vi "2D scan tiled.vi"(6 "WatchDog Mode":u16(ring)=2 items=["Do Nothing", "Send Idle Only", "Watch FIB & SEM", "Watch FIB Only", "Watch SEM Only"], 10 "Tiled scan inputs":T6={"HW Config"={"SEM X coil"="SEM-X", "SEM Y coil"="SEM-Y", "Detectors"="Detectors", "Det min (V)"=-10.0, "Det max (V)"=10.0, "Eanable COM"=TRUE, "COM port"="COM1", "Detector FIB-NI auto switch"="FIB/port0/line0", "Machine Type"=0, "Machine ID"="Feiss/Sigma-01-42", "SEM Max FOV (um)"=350.0}, "Det Info"={"Brightness A"=40.0, "Contrast A"=26.0, "Detector B name"="ESB @ 1.0 kV", "Brightness B"=40.0, "Contrast B"=40.0, "Detector C name"="PMT @ 6.0", "Detector D name"="Detector D"}, "SEM Scan Parameters"={"X size (um)"=20.0, "Y size (um)"=20.0, "X center (um)"=0.0, "Y center (um)"=0.0, "X size (V)"=6.190428211586902, "X size auto"=TRUE, "X stig"=[[0.0]], "Y stig"=[[0.0]], "X aln"=[[0.0]], "Y aln"=[[0.0]], "Scan rate (Hz)"=10000000, "Oversampling"=5, "Oversampling auto"=TRUE, "Frame line rampdown ratio"=0.1, "Pixel size (nm)"=10.0, "WD (mm)"=[[3.0]], "X tiles"=1, "Y tiles"=1, "Overlap (um)"=1.0, "Interlaced"=TRUE, "dX (um)"=[0.0], "dY (um)"=[0.0], "Frames"=1}, "SEM Options"={"GetInfo"=TRUE, "Set Det A para"=TRUE, "Set WD"=FALSE, "Set Mag"=TRUE, "Set stig"=FALSE, "Set aln"=FALSE, "Display"=TRUE, "Save"=TRUE, "8-bit"=TRUE, "Detector A"=TRUE, "Detector B"=FALSE, "Detector C"=FALSE, "Detector D"=FALSE, "Inverse A"=FALSE, "Inverse B"=FALSE, "Inverse C"=FALSE, "Inverse D"=FALSE, "Inverse PNG"=TRUE, "Freeze"=TRUE, "PNG only"=FALSE, "Upload"=FALSE, "Delete after upload"=FALSE}, "Focus Index Options"={"Keep aspect ratio"=FALSE, "Show Focus Index"=TRUE, "Focus Index primary grid center"=TRUE, "X Grids"=[[0]], "Y Grids"=[[0]], "Primary X index"=[[0]], "Primary Y index"=[[0]]}, "File Information"={"File path"=path "E:/Images", "Notes"="", "Save recipe"=FALSE, "Load recipe"=FALSE, "Sample ID"=""}, "Milling para"={"X resolution"=4096, "Y resolution"=125001, "X offset (um)"=0.0, "Y offset (um)"=0.0, "X center (um)"=0.0, "Y center (um)"=0.0, "X size (um)"=250.0, "Y size (um)"=250.0, "UL-Ang"=90.0, "UR-Ang"=90.0, "Line milling time (s)"=5.0, "Z-step (nm)"=2.0, "Lines auto pause"=1, "Auto pause"=FALSE, "Mill from Bottom"=FALSE, "FIB FOV (um)"=500.0, "Auto Profile"=FALSE, "Mill start from Last"=FALSE, "FIB PID on"=FALSE, "FIB PID reset"=TRUE, "FIB PID measured"=0, "FIB PID target"=0.0, "FIB PID target slope"=0.0, "FIB PID P"=0.001, "FIB PID I"=0.01, "FIB PID D"=0.0, "Emission (uA)"=1.36, "Suppressor (V)"=50.0, "Auto reheat"=FALSE}, "Additional Info"={"Restart flag"=0, "Stage move flag"=0}} {"Milling para"."Suppressor (V)" step=0.1 format="%.1g"; "Milling para"."Emission (uA)" step=0.1 format="%.2g"; "Milling para"."FIB PID measured" items=["Spec.", "B.D. 1", "B.D. 2", "Mill", "Spec. +"]; "Milling para"."FIB PID target slope" min=-1 max=1 step=0.1; "Milling para"."UR-Ang" format="%.2f"; "Milling para"."UL-Ang" format="%.2f"; "Milling para"."Y offset (um)" step=0.02 format="%.3g"; "Milling para"."X offset (um)" step=1 format="%.3g"; "Milling para"."FIB FOV (um)" format="%.3g"; "Milling para"."Line milling time (s)" format="%.1f"; "Milling para"."Y center (um)" format="%#.3g"; "Milling para"."X center (um)" format="%#.3g"; "SEM Scan Parameters"."dY (um)" format="%.1f"; "SEM Scan Parameters"."dX (um)" format="%.1f"; "SEM Scan Parameters"."Frames" min=1 step=1; "SEM Scan Parameters"."WD (mm)" format="%.1f"; "SEM Scan Parameters"."Y aln" format="%.1f"; "SEM Scan Parameters"."X aln" format="%.1f"; "SEM Scan Parameters"."Y stig" format="%.1f"; "SEM Scan Parameters"."X stig" format="%.1f"; "SEM Scan Parameters"."Overlap (um)" min=0; "SEM Scan Parameters"."Y tiles" min=1; "SEM Scan Parameters"."X tiles" min=1; "SEM Scan Parameters"."X size (um)" format="%.2f"; "SEM Scan Parameters"."Y size (um)" format="%.2f"; "SEM Scan Parameters"."Frame line rampdown ratio" min=0 max=1 step=0.05 format="%.2g"; "SEM Scan Parameters"."X center (um)" step=1 format="%.2f"; "SEM Scan Parameters"."Y center (um)" step=1 format="%.2f"; "SEM Scan Parameters"."X size (V)" format="%_4g"; "SEM Scan Parameters"."Scan rate (Hz)" max=4000000 step=100000 format="%.2e"; "HW Config"."Machine Type" items=["Feiss", "NVision"]}, 11 "ActiveX Container":refnum<k7>(container)) -> (0 "Image Focus Index Tiled":T3, 1 "Image Focus Index Array Tiled":T2, 2 "Low res scale Tiled (um/pix)":dbl[][](array[numeric]), 3 "Single scan outputs":T4={"SEM Status"={"AO SampClk.MaxRate"=100000000.0, "AI SampClk.MaxRate"=100000000.0, "AO rate"=10000000.0, "Scan speed"=1, "Detector #"=1, "X min (V)"=-3.095214105793451, "X max (V)"=3.095214105793451, "X min index"=0, "X max index"=1999, "AO multiline"=64, "Decimating factor"=3, "AvailSampPerChan"=832704, "AO scan line"=2000, "Total pixels recorded"=4096000, "Lines scanned"=2000, "Scan time (m)"=0.0, "Scan time (s)"=0.4416, "Remaining time (m)"=0, "Remaining time (s)"=0, "SEM Spec. I (nA)"=0.0, "Frame"=1, "X tile"=1, "Y tile"=1}, "SEM Parameters"={"Detector A"="InLens", "Detector B"="ESB @ 1.0 kV", "Brightness A"=40.0, "Contrast A"=26.0, "Brightness B"=40.0, "Contrast B"=40.0, "Magnification"=1769.4047, "Pixel size"=3.9210947, "Working distance"=2.91745, "EHT"=0.6, "Aperture"=1, "High current mode"=1, "Probe current"=613.0, "Scan rotation"=260.0, "Chamber vac"=1.43287e-06, "Gun vac"=3.9272e-10, "Beam shift X"=0.0, "Beam shift Y"=0.0, "Stig X"=-4.213583, "Stig Y"=-1.875912, "Alignment X"=1.861752, "Alignment Y"=-2.407838, "Stage X"=68.4182, "Stage Y"=64.91782, "Stage Z"=32.8349, "Stage T"=0.0, "Stage R"=153.14406, "Stage M"=0.0}, "Image Focus Index"={"A Img Focus Index"=0.014358657, "B Img Focus Index"=0.0, "C Img Focus Index"=0.0, "D Img Focus Index"=0.0}, "FIB parameters"={"FIB mode"=0, "FIB focus"=0.0, "FIB probe current"=0.0, "FIB emission current"=0.0, "FIB rotation"=0.0, "FIB aperture X"=0.0, "FIB aperture Y"=0.0, "FIB stig X"=0.0, "FIB stig Y"=0.0, "FIB beam shift X"=0.0, "FIB beam shift Y"=0.0}, "Image Focus Index Array"={"A Img Focus Index array"=[[0.014358657]], "B Img Focus Index array"=[], "C Img Focus Index array"=[], "D Img Focus Index array"=[]}} {"SEM Status"."Frame" min=1 step=1; "SEM Status"."Y tile" min=1; "SEM Status"."X tile" min=1; "SEM Status"."SEM Spec. I (nA)" format="%.2g"; "SEM Status"."AvailSampPerChan" scale=0.0..32000000.0; "SEM Status"."Scan time (s)" format="%.3f"; "SEM Status"."Total pixels recorded" scale=-1.0..37748736.0; "SEM Status"."Scan speed" scale=1.0..15.0; "SEM Status"."AO rate" format="%#_3e"}, 4 "SEM Spec. I Tiled (nA)":sgl[][](array[numeric]), 5 "8-bit over scale":bool[](array[boolean]))   [LabVIEW 2018]
uses:
  <vilib>/Analysis/baseanly.llb/Mean (DBL).vi
  <vilib>/Analysis/NI_AALBase.lvlib
panel:
  in  "Focus Index Options":T1={"Keep aspect ratio"=FALSE, "X Grids"=1, "Y Grids"=1, "Primary X index"=0, "Primary Y index"=0}
  out "Aln X Tiled":sgl[][](array[numeric])
  out "Aln Y Tiled":sgl[][](array[numeric])
  out "Stig Y Tiled":sgl[][](array[numeric])
  out "Stig X Tiled":sgl[][](array[numeric])
  out "WD Tiled":sgl[][](array[numeric])
  out "Det B Img Tiled":i16[][](graph)
  out "Det A Img Tiled":i16[][](graph)
  out "Tiled image Y index":u16[][](array[numeric])
  out "Tiled image X index":u16[][](array[numeric])
  out "Tiled image scale (um/pix)":sgl
  out "X size (V)":dbl[][](array[numeric])=[[2000.0]]
  out "Y center (um)":sgl[][](array[numeric])
  out "X center (um)":sgl[][](array[numeric])
  out "Y resolution":u32[][](array[numeric])=[[2000]]
  out "X resolution":u32[][](array[numeric])=[[2000]]
  in  "SEM Scan Parameters":T5={"X resolution"=6144, "Y resolution"=6144, "X center (um)"=0.0, "Y center (um)"=0.0, "X size (V)"=6.190428211586902, "X size auto"=TRUE, "X stig"=0.0, "Y stig"=0.0, "X aln"=0.0, "Y aln"=0.0, "Scan rate (Hz)"=10000000, "Oversampling"=5, "Oversampling auto"=TRUE, "Frame line rampdown ratio"=0.1, "Pixel size (nm)"=10.0, "WD (mm)"=0.0} {"Y aln" step=0.2 format="%.1g"; "X aln" step=0.2 format="%.1g"; "Y stig" step=0.2 format="%.1g"; "X stig" step=0.2 format="%.1g"; "WD (mm)" step=0.001 format="%.6g"; "Frame line rampdown ratio" min=0 max=1 step=0.05 format="%.2g"; "X center (um)" step=1.0 format="%.2f"; "Y center (um)" step=1.0 format="%.2f"; "X size (V)" format="%_4g"; "Scan rate (Hz)" max=4000000 step=100000 format="%.2e"}
  # "Hz"
  # "Scanning time"
  # "m"
  # "s"
  # "Remaining time"
  # "m"
  # "s"
  # "Direction"
  # "Start\nfrom"
  # "<"
  # "Grids"
  # "Primary"
  # "Recipe"
  # "Det"
  # "after"
  # "Detector A"
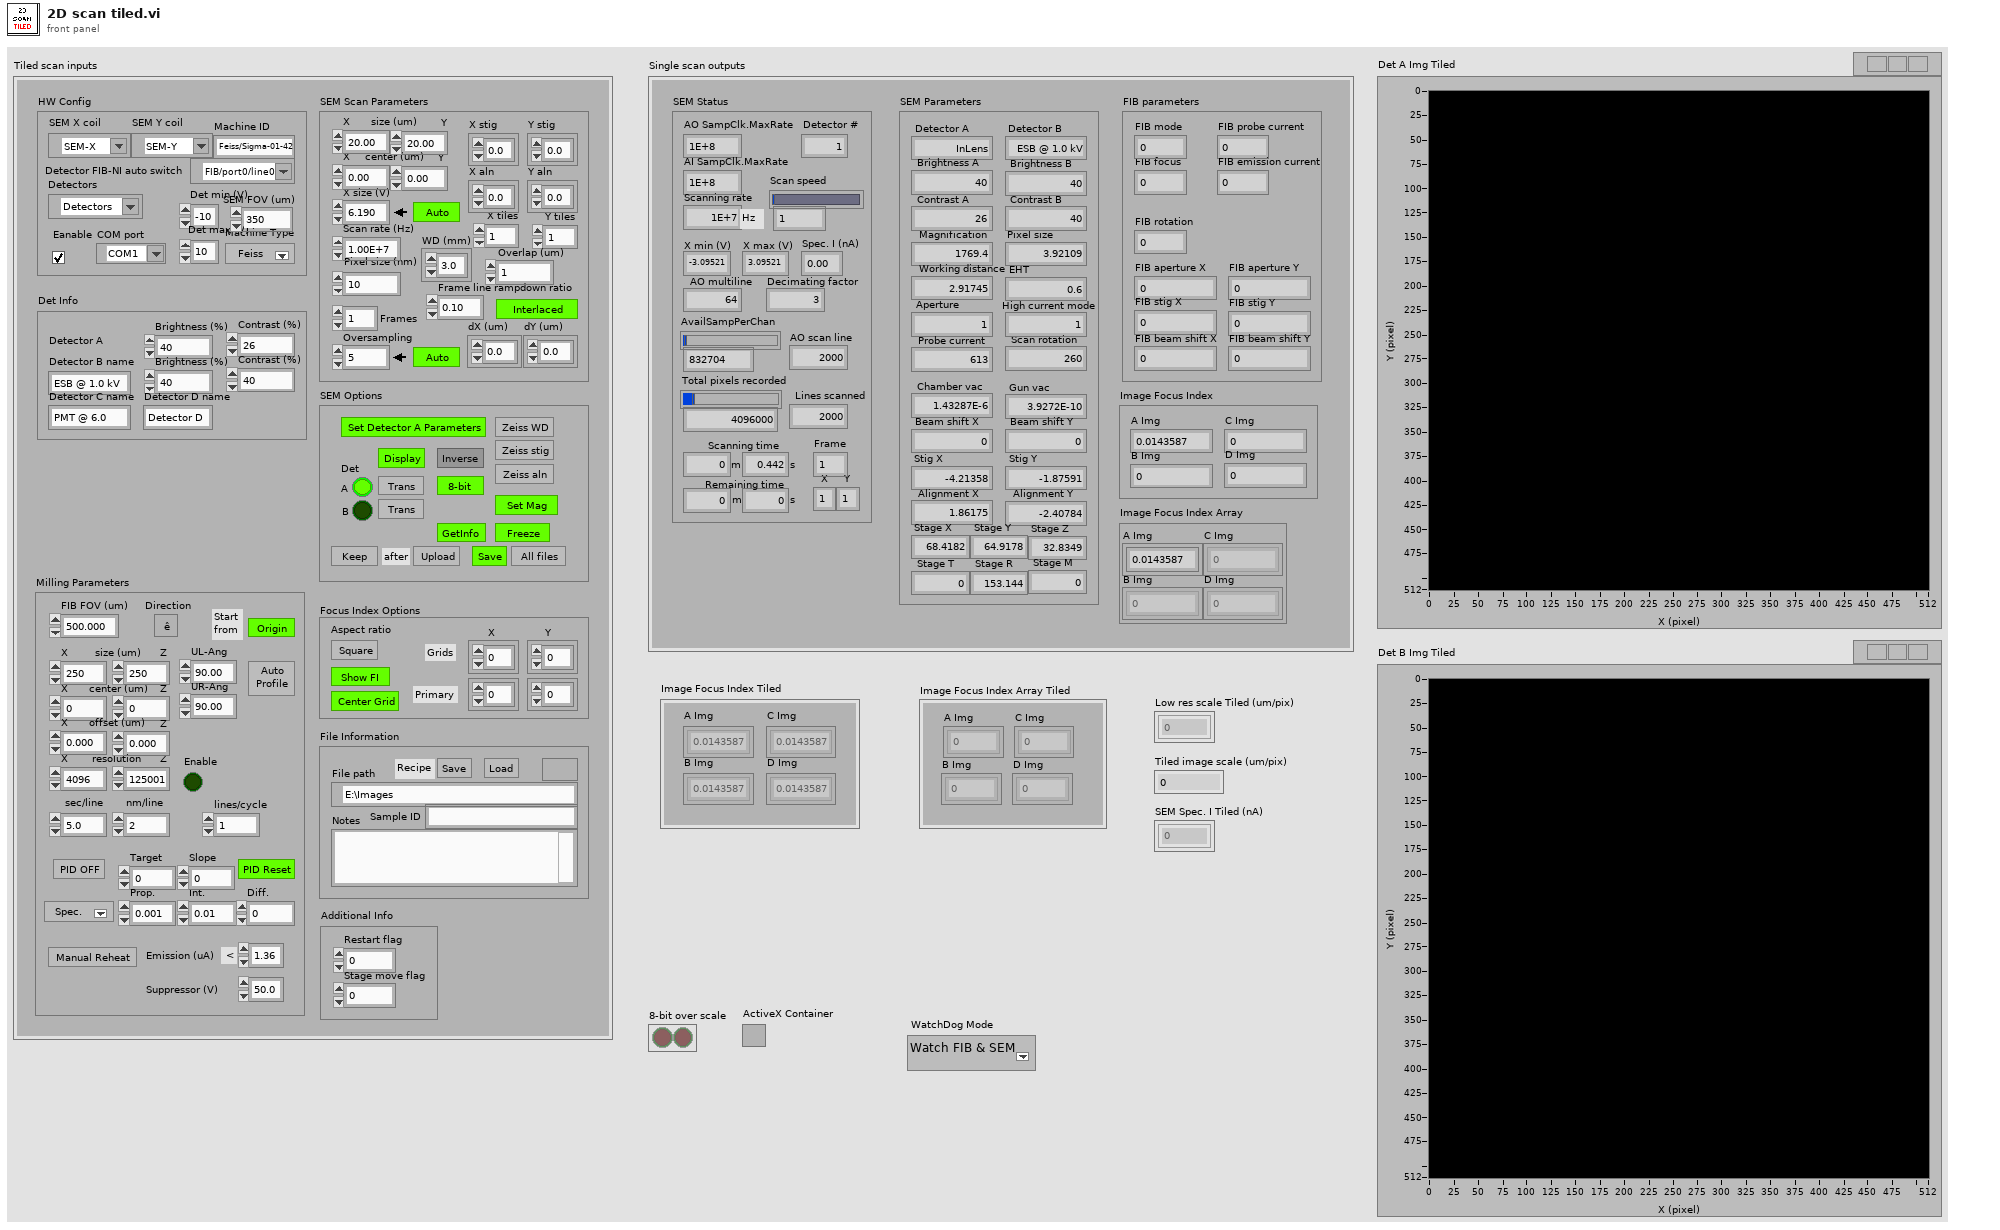
[diagram p1: front panel]
types:
  T1 = cluster{"Keep aspect ratio":bool, "X Grids":u8, "Y Grids":u8, "Primary X index":u8, "Primary Y index":u8}
  T2 = cluster{"A Img Focus Index array":sgl[][][][], "B Img Focus Index array":sgl[][][][], "C Img Focus Index array":sgl[][][][], "D Img Focus Index array":sgl[][][][]}
  T3 = cluster{"A Img Focus Index":sgl[][], "B Img Focus Index":sgl[][], "C Img Focus Index":sgl[][], "D Img Focus Index":sgl[][]}
  T4 = cluster{"SEM Status":cluster{"AO SampClk.MaxRate":dbl, "AI SampClk.MaxRate":dbl, "AO rate":dbl, "Scan speed":u8, "Detector #":u8, "X min (V)":dbl, "X max (V)":dbl, "X min index":i32, "X max index":i32, "AO multiline":u32, "Decimating factor":u16, "AvailSampPerChan":u32, "AO scan line":u32, "Total pixels recorded":i32, "Lines scanned":i32, "Scan time (m)":dbl, "Scan time (s)":dbl, "Remaining time (m)":u16, "Remaining time (s)":u8, "SEM Spec. I (nA)":sgl, "Frame":u8, "X tile":u8, "Y tile":u8}, "SEM Parameters":cluster{"Detector A":string, "Detector B":string, "Brightness A":sgl, "Contrast A":sgl, "Brightness B":sgl, "Contrast B":sgl, "Magnification":sgl, "Pixel size":sgl, "Working distance":sgl, "EHT":sgl, "Aperture":u8, "High current mode":u8, "Probe current":sgl, "Scan rotation":sgl, "Chamber vac":sgl, "Gun vac":sgl, "Beam shift X":sgl, "Beam shift Y":sgl, "Stig X":sgl, "Stig Y":sgl, "Alignment X":sgl, "Alignment Y":sgl, "Stage X":sgl, "Stage Y":sgl, "Stage Z":sgl, "Stage T":sgl, "Stage R":sgl, "Stage M":sgl}, "Image Focus Index":cluster{"A Img Focus Index":sgl, "B Img Focus Index":sgl, "C Img Focus Index":sgl, "D Img Focus Index":sgl}, "FIB parameters":cluster{"FIB mode":u8, "FIB focus":sgl, "FIB probe current":sgl, "FIB emission current":sgl, "FIB rotation":sgl, "FIB aperture X":sgl, "FIB aperture Y":sgl, "FIB stig X":sgl, "FIB stig Y":sgl, "FIB beam shift X":sgl, "FIB beam shift Y":sgl}, "Image Focus Index Array":cluster{"A Img Focus Index array":sgl[][], "B Img Focus Index array":sgl[][], "C Img Focus Index array":sgl[][], "D Img Focus Index array":sgl[][]}}
  T5 = cluster{"X resolution":u32, "Y resolution":u32, "X center (um)":dbl, "Y center (um)":dbl, "X size (V)":dbl, "X size auto":bool, "X stig":sgl, "Y stig":sgl, "X aln":sgl, "Y aln":sgl, "Scan rate (Hz)":u32, "Oversampling":u32, "Oversampling auto":bool, "Frame line rampdown ratio":sgl, "Pixel size (nm)":sgl, "WD (mm)":sgl}
  T6 = cluster{"HW Config":cluster{"SEM X coil":refnum<k15>, "SEM Y coil":refnum<k15>, "Detectors":refnum<k15>, "Det min (V)":dbl, "Det max (V)":dbl, "Eanable COM":bool, "COM port":refnum<visa-resource-name>, "Detector FIB-NI auto switch":tag, "Machine Type":u8, "Machine ID":string, "SEM Max FOV (um)":sgl}, "Det Info":cluster{"Brightness A":dbl, "Contrast A":dbl, "Detector B name":string, "Brightness B":dbl, "Contrast B":dbl, "Detector C name":string, "Detector D name":string}, "SEM Scan Parameters":cluster{"X size (um)":sgl, "Y size (um)":sgl, "X center (um)":sgl, "Y center (um)":sgl, "X size (V)":dbl, "X size auto":bool, "X stig":sgl[][], "Y stig":sgl[][], "X aln":sgl[][], "Y aln":sgl[][], "Scan rate (Hz)":u32, "Oversampling":u32, "Oversampling auto":bool, "Frame line rampdown ratio":sgl, "Pixel size (nm)":sgl, "WD (mm)":sgl[][], "X tiles":u8, "Y tiles":u8, "Overlap (um)":sgl, "Interlaced":bool, "dX (um)":sgl[], "dY (um)":sgl[], "Frames":u8}, "SEM Options":cluster{"GetInfo":bool, "Set Det A para":bool, "Set WD":bool, "Set Mag":bool, "Set stig":bool, "Set aln":bool, "Display":bool, "Save":bool, "8-bit":bool, "Detector A":bool, "Detector B":bool, "Detector C":bool, "Detector D":bool, "Inverse A":bool, "Inverse B":bool, "Inverse C":bool, "Inverse D":bool, "Inverse PNG":bool, "Freeze":bool, "PNG only":bool, "Upload":bool, "Delete after upload":bool}, "Focus Index Options":cluster{"Keep aspect ratio":bool, "Show Focus Index":bool, "Focus Index primary grid center":bool, "X Grids":u8[][], "Y Grids":u8[][], "Primary X index":u8[][], "Primary Y index":u8[][]}, "File Information":cluster{"File path":path, "Notes":string, "Save recipe":bool, "Load recipe":bool, "Sample ID":string}, "Milling para":cluster{"X resolution":u32, "Y resolution":u32, "X offset (um)":sgl, "Y offset (um)":sgl, "X center (um)":sgl, "Y center (um)":sgl, "X size (um)":sgl, "Y size (um)":sgl, "UL-Ang":sgl, "UR-Ang":sgl, "Line milling time (s)":sgl, "Z-step (nm)":dbl, "Lines auto pause":u16, "Auto pause":bool, "Mill from Bottom":bool, "FIB FOV (um)":sgl, "Auto Profile":bool, "Mill start from Last":bool, "FIB PID on":bool, "FIB PID reset":bool, "FIB PID measured":u8, "FIB PID target":sgl, "FIB PID target slope":sgl, "FIB PID P":sgl, "FIB PID I":sgl, "FIB PID D":sgl, "Emission (uA)":dbl, "Suppressor (V)":sgl, "Auto reheat":bool}, "Additional Info":cluster{"Restart flag":u8, "Stage move flag":u8}}
  T7 = cluster{"GetInfo":bool, "Set Det A para":bool, "Set WD":bool, "Set Mag":bool, "Set stig":bool, "Set aln":bool, "Display":bool, "Save":bool, "8-bit":bool, "Detector A":bool, "Detector B":bool, "Detector C":bool, "Detector D":bool, "Inverse A":bool, "Inverse B":bool, "Inverse C":bool, "Inverse D":bool, "Inverse PNG":bool, "Freeze":bool, "PNG only":bool, "Upload":bool, "Delete after upload":bool}
  T8 = cluster{"SEM X coil":refnum<k15>, "SEM Y coil":refnum<k15>, "Detectors":refnum<k15>, "Det min (V)":dbl, "Det max (V)":dbl, "Eanable COM":bool, "COM port":refnum<visa-resource-name>, "Detector FIB-NI auto switch":tag, "Machine Type":u8, "Machine ID":string, "SEM Max FOV (um)":sgl}
  T9 = cluster{"Brightness A":dbl, "Contrast A":dbl, "Detector B name":string, "Brightness B":dbl, "Contrast B":dbl, "Detector C name":string, "Detector D name":string}
  T10 = cluster{"X size (um)":sgl, "Y size (um)":sgl, "X center (um)":sgl, "Y center (um)":sgl, "X size (V)":dbl, "X size auto":bool, "X stig":sgl[][], "Y stig":sgl[][], "X aln":sgl[][], "Y aln":sgl[][], "Scan rate (Hz)":u32, "Oversampling":u32, "Oversampling auto":bool, "Frame line rampdown ratio":sgl, "Pixel size (nm)":sgl, "WD (mm)":sgl[][], "X tiles":u8, "Y tiles":u8, "Overlap (um)":sgl, "Interlaced":bool, "dX (um)":sgl[], "dY (um)":sgl[], "Frames":u8}
  T11 = cluster{"Keep aspect ratio":bool, "Show Focus Index":bool, "Focus Index primary grid center":bool, "X Grids":u8[][], "Y Grids":u8[][], "Primary X index":u8[][], "Primary Y index":u8[][]}
  T12 = cluster{"File path":path, "Notes":string, "Save recipe":bool, "Load recipe":bool, "Sample ID":string}
  T13 = cluster{"X resolution":u32, "Y resolution":u32, "X offset (um)":sgl, "Y offset (um)":sgl, "X center (um)":sgl, "Y center (um)":sgl, "X size (um)":sgl, "Y size (um)":sgl, "UL-Ang":sgl, "UR-Ang":sgl, "Line milling time (s)":sgl, "Z-step (nm)":dbl, "Lines auto pause":u16, "Auto pause":bool, "Mill from Bottom":bool, "FIB FOV (um)":sgl, "Auto Profile":bool, "Mill start from Last":bool, "FIB PID on":bool, "FIB PID reset":bool, "FIB PID measured":u8, "FIB PID target":sgl, "FIB PID target slope":sgl, "FIB PID P":sgl, "FIB PID I":sgl, "FIB PID D":sgl, "Emission (uA)":dbl, "Suppressor (V)":sgl, "Auto reheat":bool}
  T14 = cluster{"A Img Focus Index array":sgl[][], "B Img Focus Index array":sgl[][], "C Img Focus Index array":sgl[][], "D Img Focus Index array":sgl[][]}
  T15 = cluster{"AO SampClk.MaxRate":dbl, "AI SampClk.MaxRate":dbl, "AO rate":dbl, "Scan speed":u8, "Detector number":u8, "X min (V)":dbl, "X max (V)":dbl, "X min index":i32, "X max index":i32, "AO multiline":u32, "Decimating factor":u16, "AvailSampPerChan":u32, "AO scan line":u32, "Total pixels recorded":i32, "Total lines scanned":i32, "Scan time (m)":dbl, "Scan time (s)":dbl, "Remaining time (m)":u16, "Remaining time (s)":u8, "Specimen I (nA)":sgl, "Frame":u8, "X tile":u8, "Y tile":u8}
  T16 = cluster{"Detector A":string, "Detector B":string, "Brightness A":sgl, "Contrast A":sgl, "Brightness B":sgl, "Contrast B":sgl, "Magnification":sgl, "Pixel size":sgl, "Working distance":sgl, "EHT":sgl, "Aperture":u8, "High current mode":u8, "Probe current":sgl, "Scan rotation":sgl, "Chamber vac":sgl, "Gun vac":sgl, "Beam shift X":sgl, "Beam shift Y":sgl, "Stig X":sgl, "Stig Y":sgl, "Alignment X":sgl, "Alignment Y":sgl, "Stage X":sgl, "Stage Y":sgl, "Stage Z":sgl, "Stage T":sgl, "Stage R":sgl, "Stage M":sgl}
  T17 = cluster{"FIB mode":u8, "FIB focus":sgl, "FIB probe current":sgl, "FIB emission current":sgl, "FIB rotation":sgl, "FIB aperture X":sgl, "FIB aperture Y":sgl, "FIB stig X":sgl, "FIB stig Y":sgl, "FIB beam shift X":sgl, "FIB beam shift Y":sgl}
  T18 = cluster{"A Img Focus Index":sgl, "B Img Focus Index":sgl, "C Img Focus Index":sgl, "D Img Focus Index":sgl}
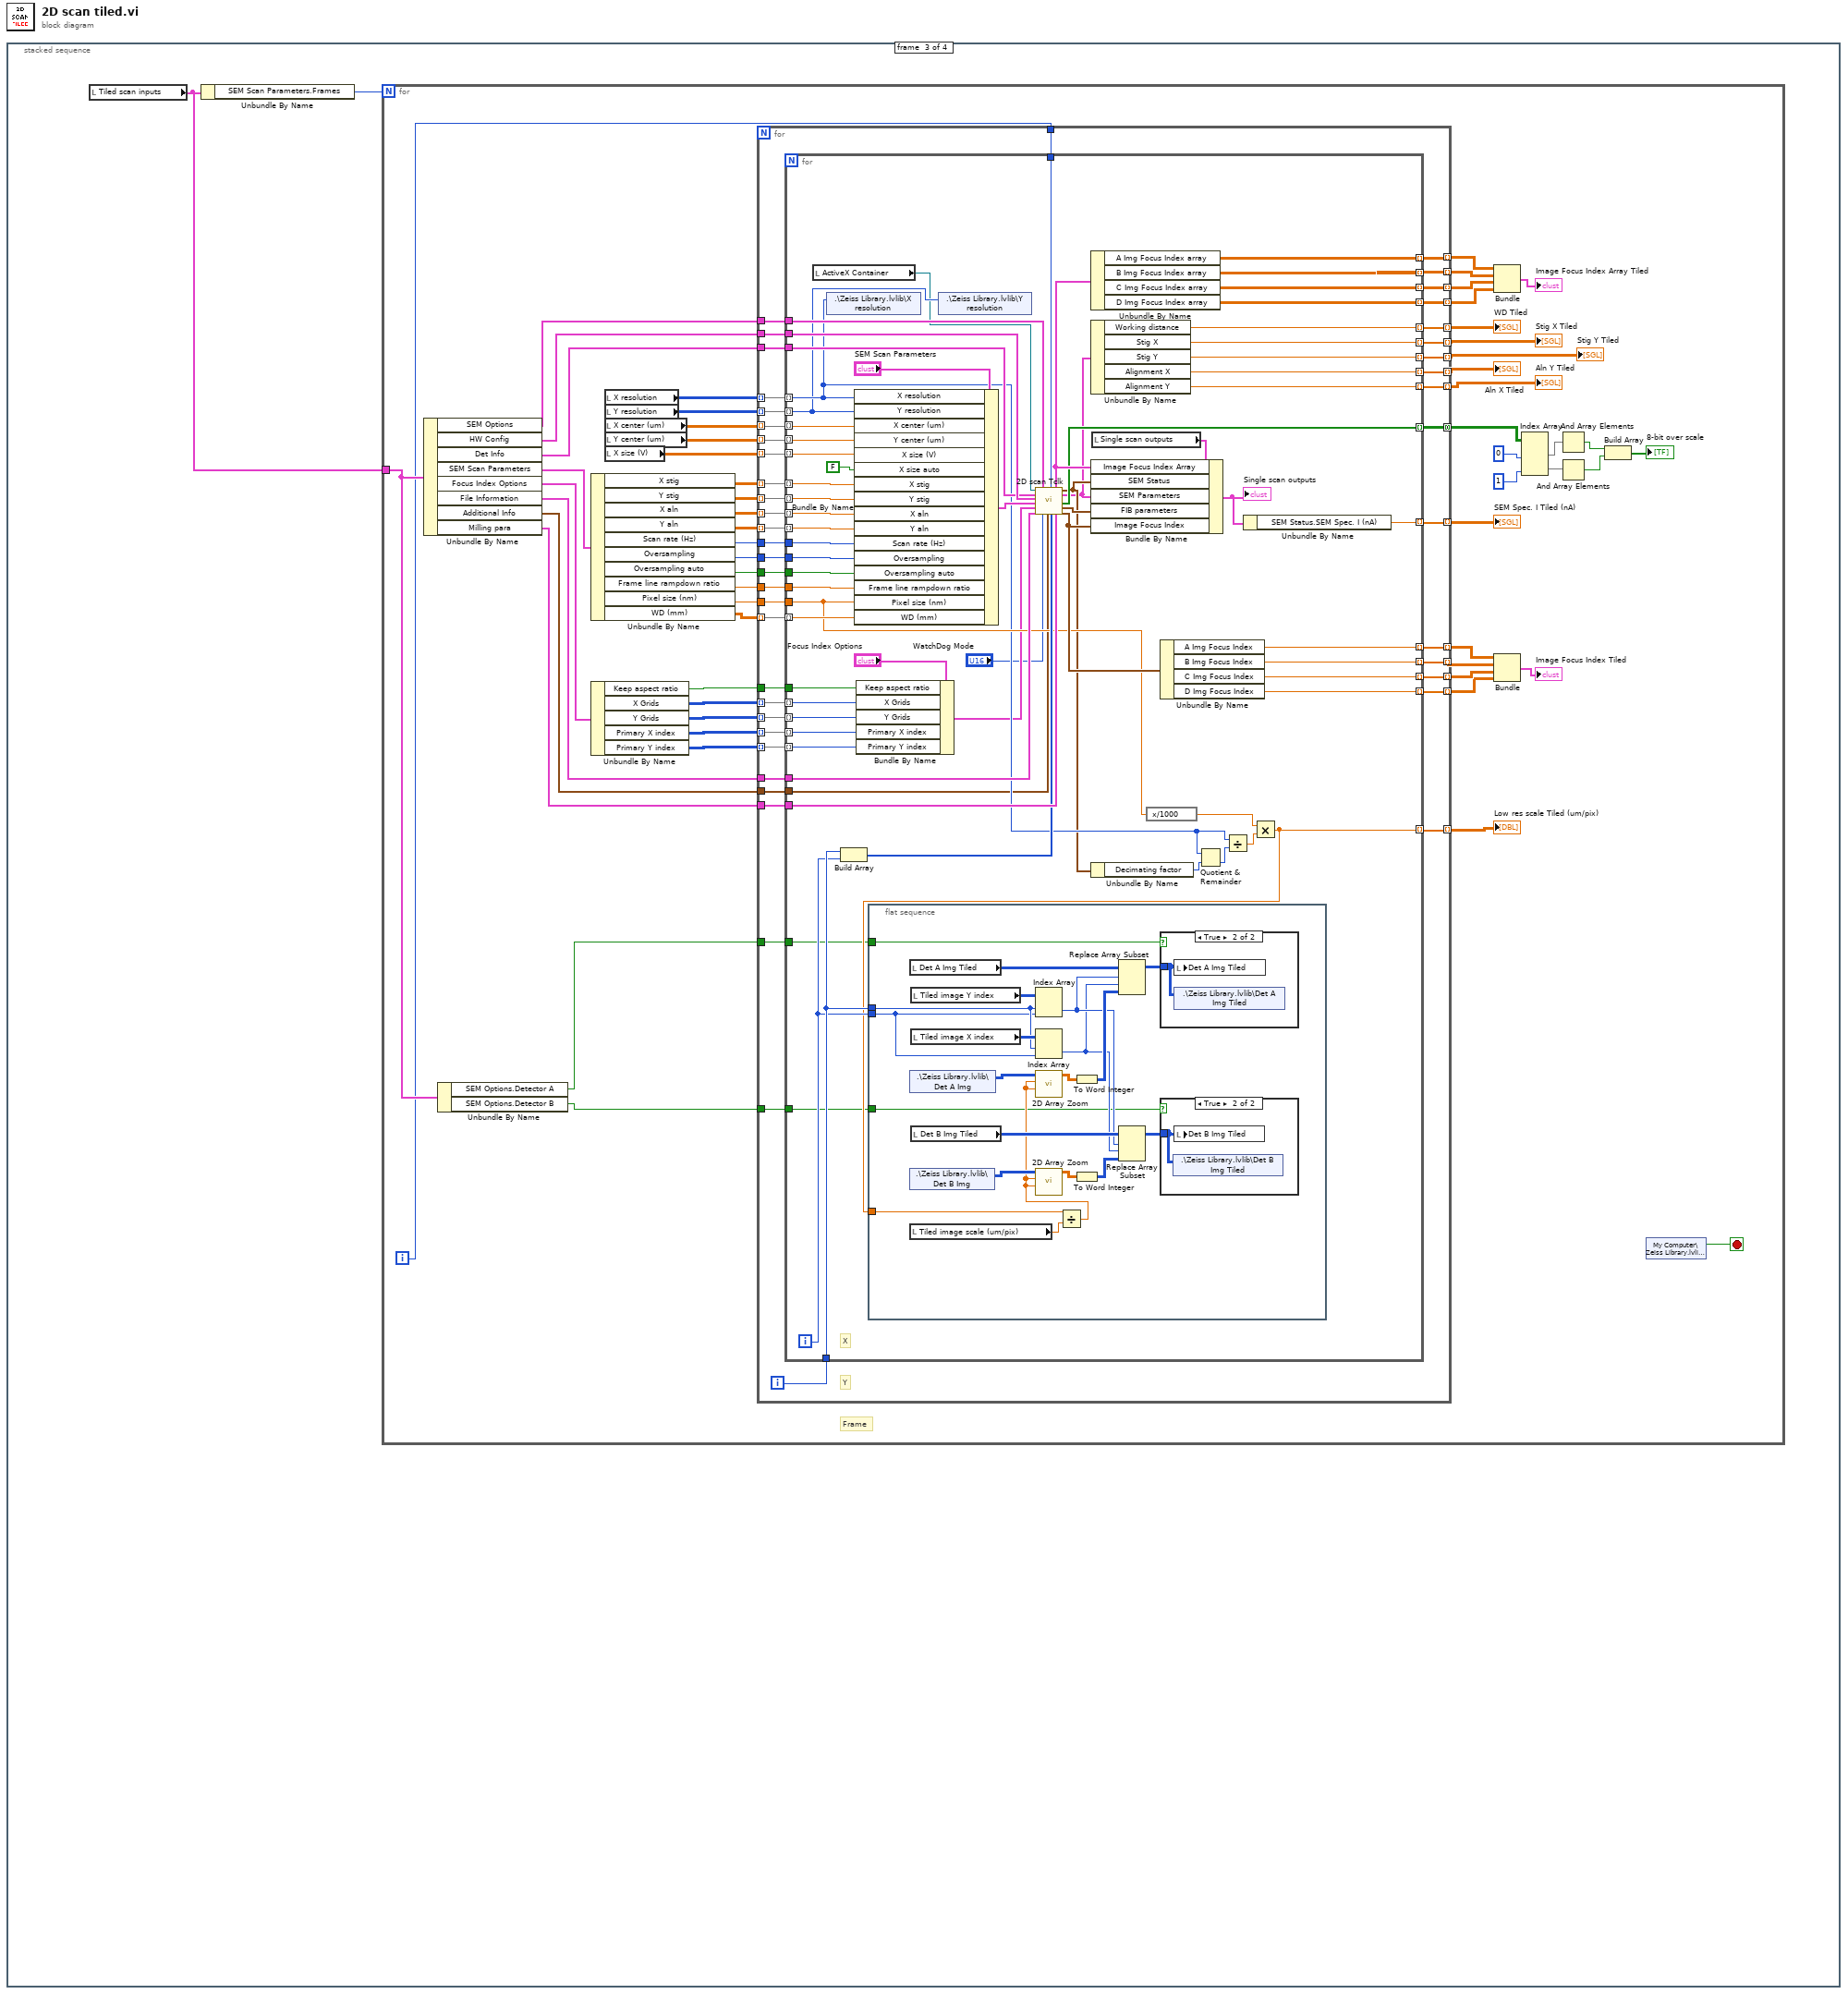
[diagram p0: block diagram]
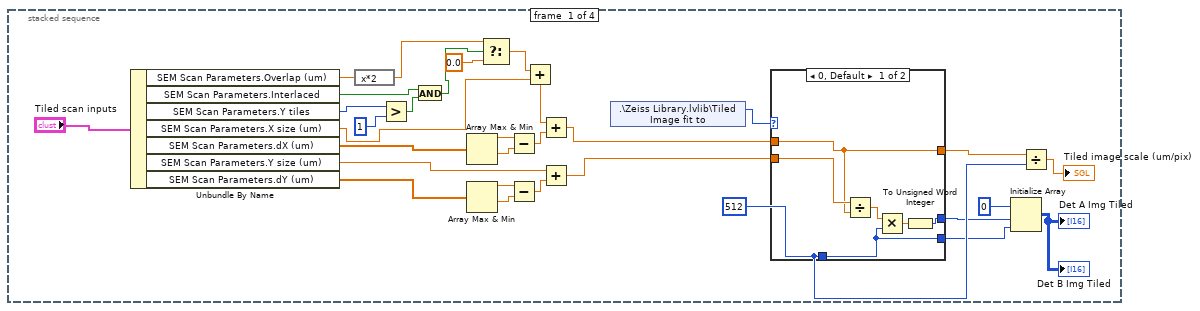
[diagram p2: hidden frame]
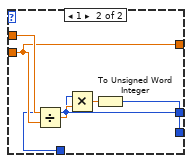
[diagram p3: hidden frame]
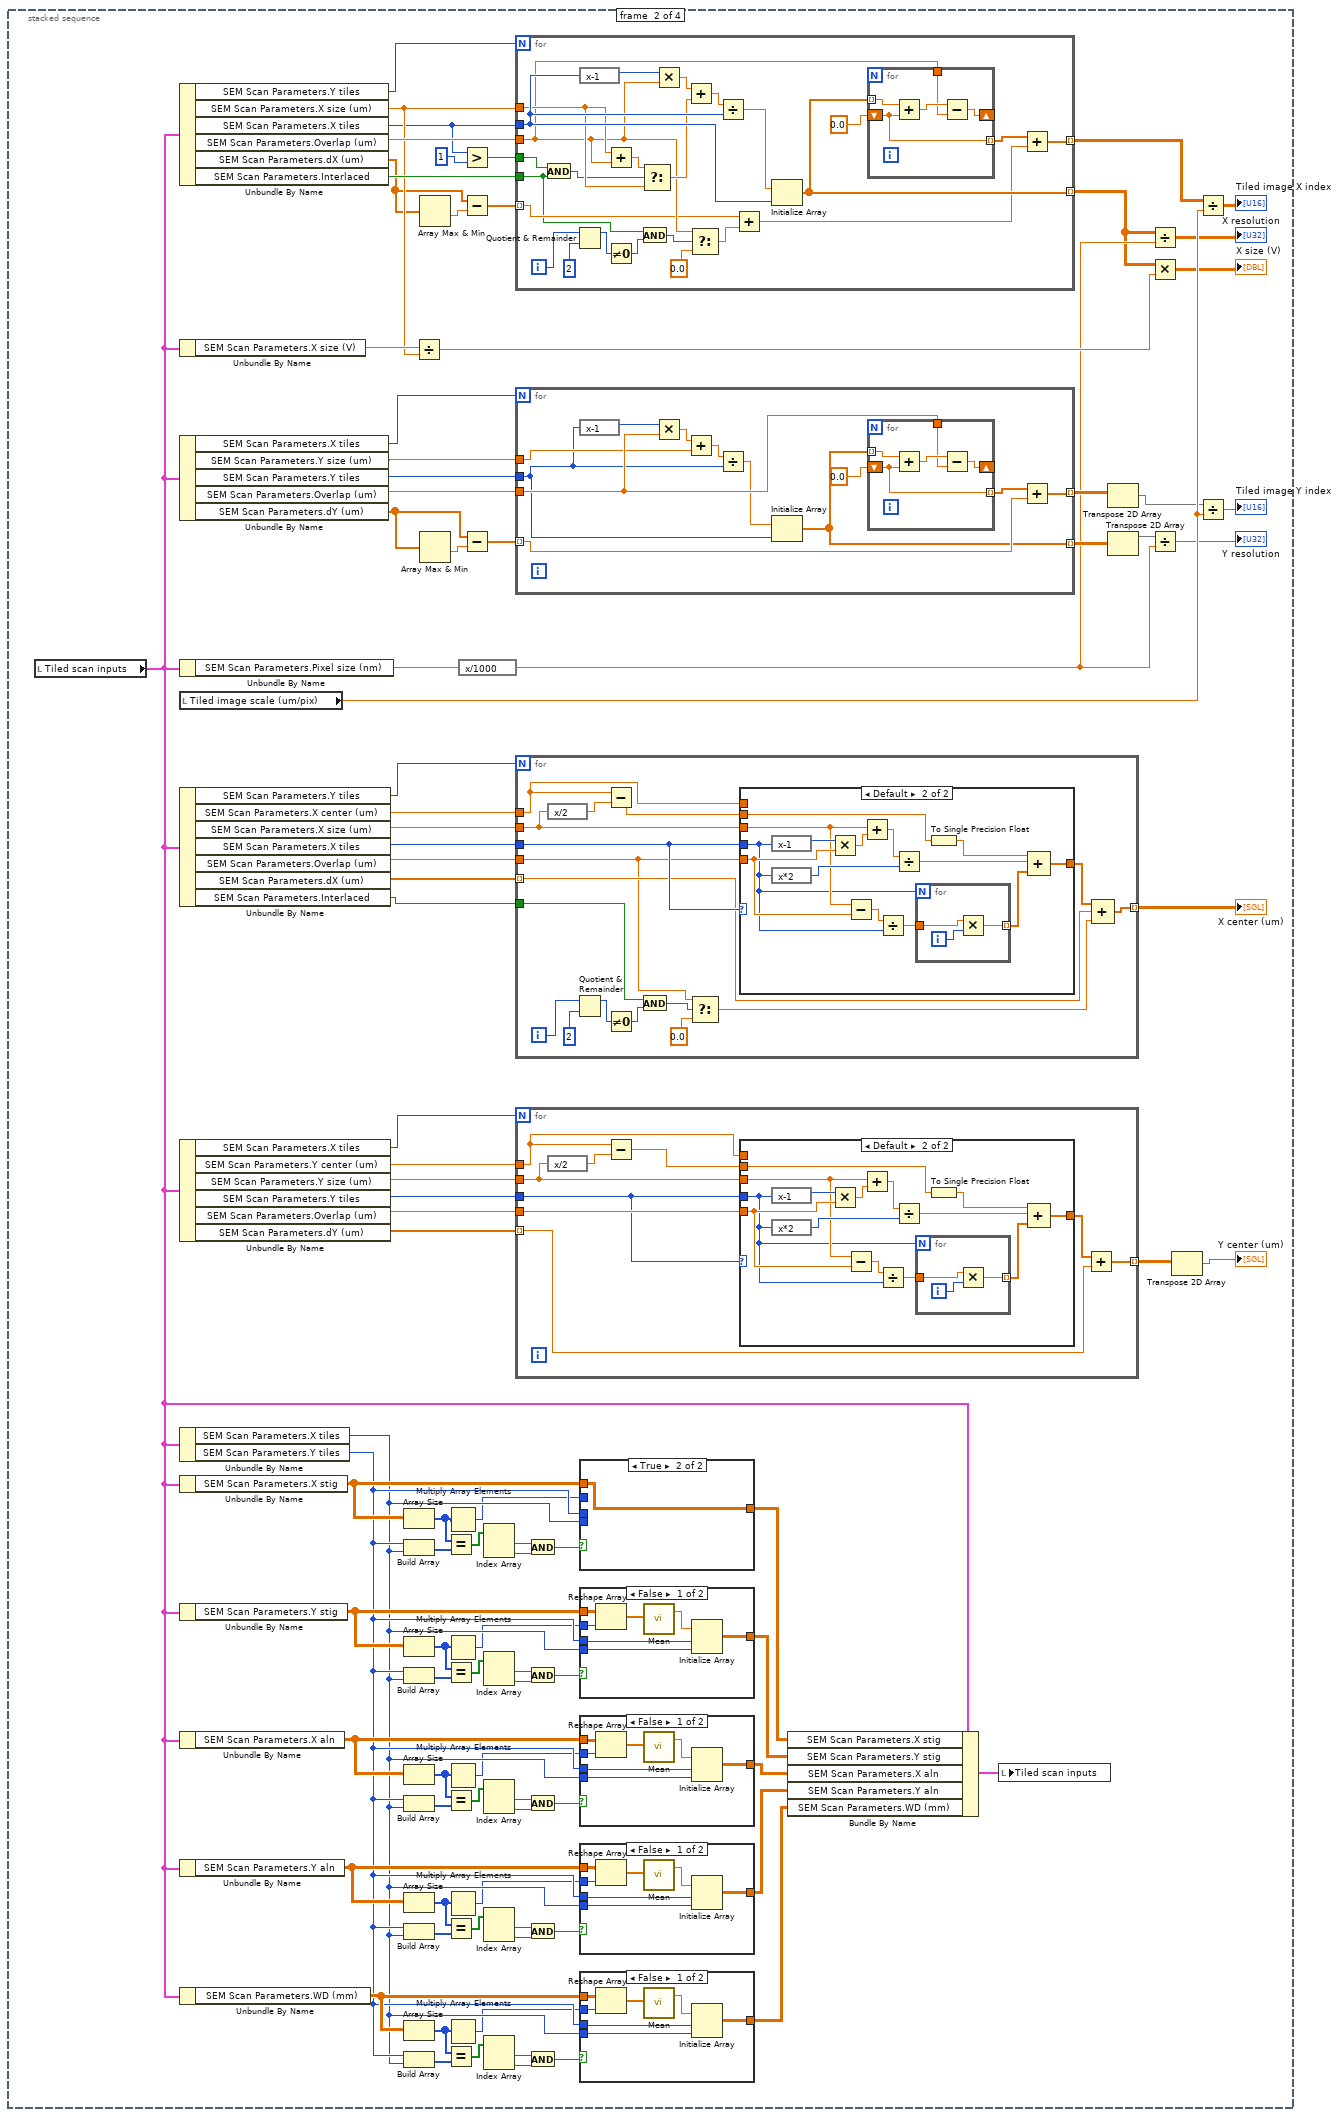
[diagram p4: hidden frame]
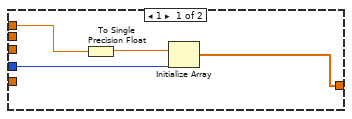
[diagram p5: hidden frame]
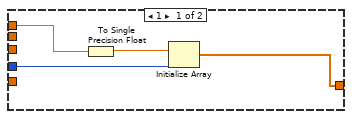
[diagram p6: hidden frame]
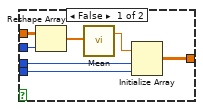
[diagram p11: hidden frame]
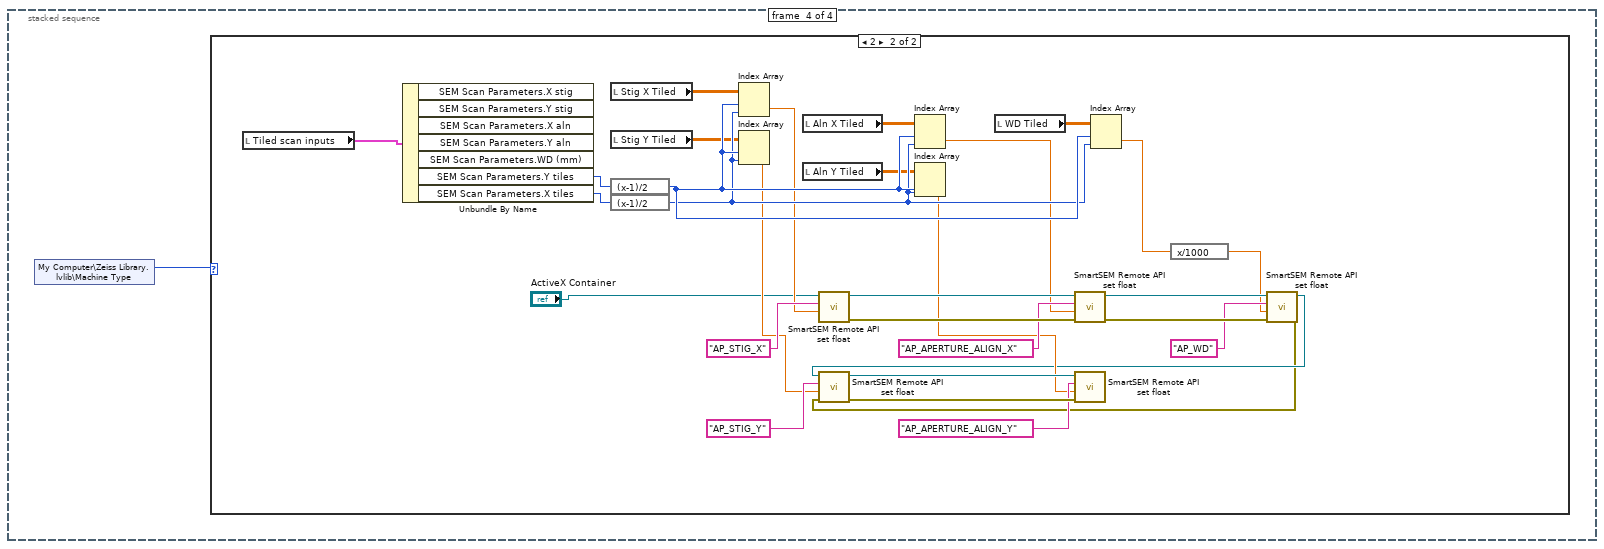
[diagram p14: hidden frame]
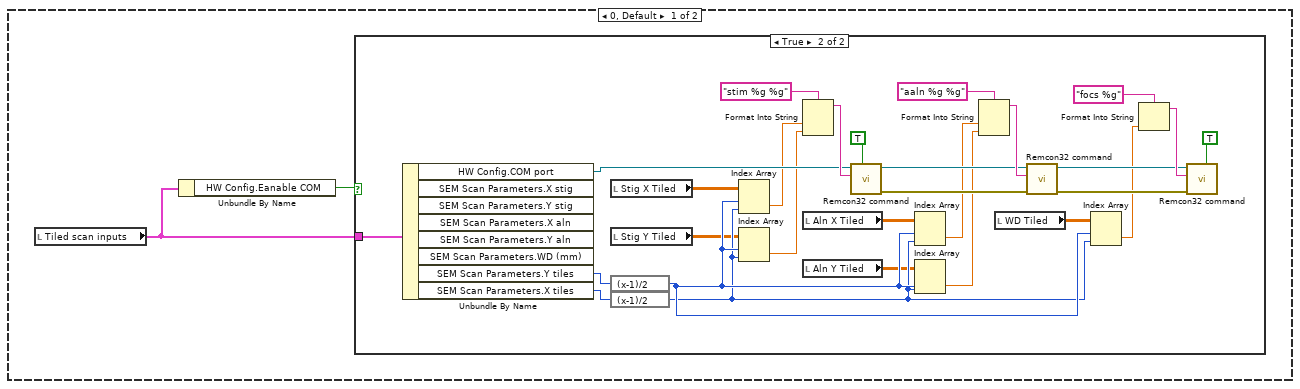
[diagram p15: hidden frame]
diagram:
  n1 = stacked-sequence {
    frame #0 {
      w28 = u16 512 ("y")
      n2 = Unbundle By Name("Tiled scan inputs") -> ("SEM Scan Parameters.Overlap (um)"=w7:sgl, "SEM Scan Parameters.Interlaced"=w2:bool, "SEM Scan Parameters.Y tiles"=w5:u8, "SEM Scan Parameters.X size (um)"=w10:sgl, "SEM Scan Parameters.dX (um)"=w22:sgl[], "SEM Scan Parameters.Y size (um)"=w13:sgl, "SEM Scan Parameters.dY (um)"=w14:sgl[])
      n3 = expression code="x*2"(w7) -> (w6:sgl)
      n4 = Greater?(x=w5, y=u8 1) -> (0:w3:bool)
      n5 = And(x=w2, y=w3) -> (x .and. y?=w1:bool)
      n6 = Array Max & Min(array=w22) -> (max value=w21:sgl, min value=w20:sgl)  [unwired: 2 out]
      n7 = Array Max & Min(array=w14) -> (max value=w15:sgl, min value=w16:sgl)  [unwired: 2 out]
      n8 = Select(t=w6, s=w1, f=0.0) -> (s? t:f=w9:dbl)
      n9 = Subtract(x=w21, y=w20) -> (x-y=w19:sgl)
      n10 = Subtract(x=w15, y=w16) -> (x-y=w17:sgl)
      n11 = Add(x=w9, y=w10) -> (x+y=w11:dbl)
      n12 = Add(x=w11, y=w19) -> (x+y=w18:dbl)
      n13 = Add(x=w13, y=w17) -> (x+y=w12:sgl)
      n14 = shared-variable ".\\Zeiss Library.lvlib\\Tiled Image fit to"() -> (w23:u8)  [unwired: 1 in, 1 out]
      n15 = case shown="0, Default" w23 {
        tunnel: w18 -> [w36 w42]
        tunnel: w12 -> [w37 w41]
        tunnel: [w36 w41] -> w29
        tunnel: w28 -> [w34 w39]
        tunnel: [w34 w38] -> w26
        tunnel: [w32 w39] -> w27
        frame 0, Default {
          n16 = Divide(x=w37, y=w36) -> (x/y=w35:dbl)
          n17 = Multiply(x=w35, y=w34) -> (x*y=w33:dbl)
          n18 = To Unsigned Word Integer(number=w33) -> (unsigned 16bit integer=w32:u16)
        }
        frame 1 {
          n19 = Divide(x=w42, y=w41) -> (x/y=w40:dbl)
          n20 = Multiply(x=w39, y=w40) -> (x*y=w43:dbl)
          n21 = To Unsigned Word Integer(number=w43) -> (unsigned 16bit integer=w38:u16)
        }
      }
      n22 = Initialize Array(i16 0 ("element"), w27, w26) -> (→"Det A Img Tiled" →"Det B Img Tiled":i16[][])
      n23 = Divide(x=w29, y=w28) -> (x/y=→"Tiled image scale (um/pix)":dbl)
    }
    frame #1 {
      n24 = local read "Tiled scan inputs"() -> (w68:T6)
      n25 = Unbundle By Name(w68) -> ("SEM Scan Parameters.Y tiles"=w60:u8, "SEM Scan Parameters.X size (um)"=w69:sgl, "SEM Scan Parameters.X tiles"=w46:u8, "SEM Scan Parameters.Overlap (um)"=w135:sgl, "SEM Scan Parameters.dX (um)"=w57:sgl[], "SEM Scan Parameters.Interlaced"=w128:bool)
      n26 = Unbundle By Name(w68) -> ("SEM Scan Parameters.X size (V)"=w70:dbl)
      n27 = Unbundle By Name(w68) -> ("SEM Scan Parameters.X tiles"=w130:u8, "SEM Scan Parameters.Y size (um)"=w131:sgl, "SEM Scan Parameters.Y tiles"=w133:u8, "SEM Scan Parameters.Overlap (um)"=w132:sgl, "SEM Scan Parameters.dY (um)"=w53:sgl[])
      n28 = Unbundle By Name(w68) -> ("SEM Scan Parameters.Pixel size (nm)"=w134:sgl)
      n29 = local read "Tiled image scale (um/pix)"() -> (w66:sgl)
      n30 = Unbundle By Name(w68) -> ("SEM Scan Parameters.Y tiles"=w59:u8, "SEM Scan Parameters.X center (um)"=w122:sgl, "SEM Scan Parameters.X size (um)"=w123:sgl, "SEM Scan Parameters.X tiles"=w126:u8, "SEM Scan Parameters.Overlap (um)"=w124:sgl, "SEM Scan Parameters.dX (um)"=w125:sgl[], "SEM Scan Parameters.Interlaced"=w127:bool)
      n31 = Unbundle By Name(w68) -> ("SEM Scan Parameters.X tiles"=w115:u8, "SEM Scan Parameters.Y center (um)"=w120:sgl, "SEM Scan Parameters.Y size (um)"=w119:sgl, "SEM Scan Parameters.Y tiles"=w116:u8, "SEM Scan Parameters.Overlap (um)"=w118:sgl, "SEM Scan Parameters.dY (um)"=w117:sgl[])
      n32 = Unbundle By Name(w68) -> ("SEM Scan Parameters.X tiles"=w84:u8, "SEM Scan Parameters.Y tiles"=w85:u8)
      n33 = Unbundle By Name(w68) -> ("SEM Scan Parameters.X stig"=w141:sgl[][])
      n34 = Unbundle By Name(w68) -> ("SEM Scan Parameters.Y stig"=w102:sgl[][])
      n35 = Unbundle By Name(w68) -> ("SEM Scan Parameters.X aln"=w88:sgl[][])
      n36 = Unbundle By Name(w68) -> ("SEM Scan Parameters.Y aln"=w87:sgl[][])
      n37 = Unbundle By Name(w68) -> ("SEM Scan Parameters.WD (mm)"=w86:sgl[][])
      n38 = Array Size(array=w141) -> (size(s)=w80:i32[])
      n39 = Build Array(w85, w84) -> (w111:u8[])
      n40 = Array Size(array=w102) -> (size(s)=w75:i32[])
      n41 = Build Array(w85, w84) -> (w103:u8[])
      n42 = Array Size(array=w88) -> (size(s)=w76:i32[])
      n43 = Build Array(w85, w84) -> (w100:u8[])
      n44 = Array Size(array=w87) -> (size(s)=w78:i32[])
      n45 = Build Array(w85, w84) -> (w93:u8[])
      n46 = Array Size(array=w86) -> (size(s)=w77:i32[])
      n47 = Build Array(w85, w84) -> (w92:u8[])
      n48 = Divide(x=w70, y=w69) -> (x/y=w51:dbl)
      n49 = Array Max & Min(array=w57) -> (min value=w58:sgl)  [unwired: 3 out]
      n50 = Array Max & Min(array=w53) -> (min value=w55:sgl)  [unwired: 3 out]
      n51 = Equal?(x=w80, y=w111) -> (x = y?=w110:bool[])
      n52 = Equal?(x=w75, y=w103) -> (x = y?=w104:bool[])
      n53 = Equal?(x=w76, y=w100) -> (x = y?=w99:bool[])
      n54 = Equal?(x=w78, y=w93) -> (x = y?=w94:bool[])
      n55 = Equal?(x=w77, y=w92) -> (x = y?=w91:bool[])
      n56 = Multiply Array Elements(1:w80) -> (0:w79:i32)
      n57 = Multiply Array Elements(1:w75) -> (0:w74:i32)
      n58 = Multiply Array Elements(1:w76) -> (0:w73:i32)
      n59 = Multiply Array Elements(1:w78) -> (0:w72:i32)
      n60 = Multiply Array Elements(1:w77) -> (0:w71:i32)
      n61 = expression code="x/1000"(w134) -> (w50:sgl)
      n62 = Greater?(x=w46, y=u8 1) -> (0:w44:bool)
      n63 = Subtract(x=w57, y=w58) -> (x-y=w56:sgl[])
      n64 = Subtract(x=w53, y=w55) -> (x-y=w54:sgl[])
      n65 = Index Array(array=w110) -> (element #1=w108:bool, element #2=w109:bool)  [unwired: 2 in]
      n66 = Index Array(array=w104) -> (element #1=w106:bool, element #2=w105:bool)  [unwired: 2 in]
      n67 = Index Array(array=w99) -> (element #1=w97:bool, element #2=w98:bool)  [unwired: 2 in]
      n68 = Index Array(array=w94) -> (element #1=w96:bool, element #2=w95:bool)  [unwired: 2 in]
      n69 = Index Array(array=w91) -> (element #1=w89:bool, element #2=w90:bool)  [unwired: 2 in]
      n70 = for {
        N: w60 -> [_]
        tunnel: w69 -> [w241]
        tunnel: w135 -> [w236]
        tunnel: w46 -> [w247]
        tunnel: [w251] -> w48 mode=indexing
        tunnel: w128 -> [w229]
        tunnel: [w243] -> w63 mode=indexing
        tunnel: w56 -> [w233] mode=indexing
        tunnel: w44 -> [w228]
        i -> [w237]
        n71 = And(x=w228, y=w229) -> (x .and. y?=w227:bool)
        n72 = Quotient & Remainder(x=w237, y=2) -> (x-y*floor(x/y)=w239:i32)  [unwired: 1 out]
        n73 = expression code="x-1"(w247) -> (w245:u8)
        n74 = Add(x=w241, y=w236) -> (x+y=w242:sgl)
        n75 = Not Equal To 0?(x=w239) -> (x != 0?=w231:bool)
        n76 = And(x=w229, y=w231) -> (x .and. y?=w230:bool)
        n77 = Select(t=w242, s=w227, f=w241) -> (s? t:f=w240:sgl)
        n78 = Multiply(x=w245, y=w236) -> (x*y=w249:sgl)
        n79 = Add(x=w249, y=w240) -> (x+y=w248:sgl)
        n80 = Select(t=w236, s=w230, f=sgl 0.0) -> (s? t:f=w234:sgl)
        n81 = Divide(x=w248, y=w247) -> (x/y=w246:sgl)
        n82 = Add(x=w233, y=w234) -> (x+y=w232:sgl)
        n83 = Initialize Array(w246, w247) -> (w251:sgl[])
        n84 = for {
          tunnel: w251 -> [w256] mode=indexing
          shift-right: [w253] -> _
          shift-left: sgl 0.0 -> [w254]
          tunnel: [w254] -> w244 mode=indexing
          tunnel: w236 -> [w252]
          n85 = Add(x=w256, y=w254) -> (x+y=w255:sgl)
          n86 = Subtract(x=w255, y=w252) -> (x-y=w253:sgl)
        }
        n87 = Add(x=w244, y=w232) -> (x+y=w243:sgl[])
      }
      n88 = for {
        N: w130 -> [_]
        tunnel: w133 -> [w143]
        tunnel: w132 -> [w146]
        tunnel: w131 -> [w145]
        tunnel: [w142] -> w129 mode=indexing
        tunnel: [w151] -> w62 mode=indexing
        tunnel: w54 -> [w150] mode=indexing
        n89 = expression code="x-1"(w143) -> (w149:u8)
        n90 = Multiply(x=w149, y=w146) -> (x*y=w147:sgl)
        n91 = Add(x=w147, y=w145) -> (x+y=w148:sgl)
        n92 = Divide(x=w148, y=w143) -> (x/y=w144:sgl)
        n93 = Initialize Array(w144, w143) -> (w142:sgl[])
        n94 = for {
          tunnel: w142 -> [w158] mode=indexing
          shift-right: [w155] -> _
          shift-left: sgl 0.0 -> [w156]
          tunnel: [w156] -> w152 mode=indexing
          tunnel: w146 -> [w154]
          n95 = Add(x=w158, y=w156) -> (x+y=w157:sgl)
          n96 = Subtract(x=w157, y=w154) -> (x-y=w155:sgl)
        }
        n97 = Add(x=w152, y=w150) -> (x+y=w151:sgl[])
      }
      n98 = for {
        N: w59 -> [_]
        tunnel: w123 -> [w204]
        tunnel: w124 -> [w189]
        tunnel: w125 -> [w190] mode=indexing
        tunnel: w126 -> [w205]
        tunnel: [w192] -> w121 mode=indexing
        tunnel: w127 -> [w196]
        tunnel: w122 -> [w201]
        i -> [w197]
        n99 = expression code="x/2"(w204) -> (w203:sgl)
        n100 = Quotient & Remainder(x=w197, y=2) -> (x-y*floor(x/y)=w200:i32)  [unwired: 1 out]
        n101 = Subtract(x=w201, y=w203) -> (x-y=w202:sgl)
        n102 = Not Equal To 0?(x=w200) -> (x != 0?=w199:bool)
        n103 = And(x=w196, y=w199) -> (x .and. y?=w194:bool)
        n104 = Select(t=w189, s=w194, f=sgl 0.0) -> (s? t:f=w191:sgl)
        n105 = case shown="Default" w205 {
          tunnel: w204 -> [_ w216]
          tunnel: w189 -> [_ w217]
          tunnel: w205 -> [w209 w214]
          tunnel: [w208 w211] -> w193
          tunnel: w202 -> [_ w218]
          tunnel: w201 -> [w207 _]
          frame 1 {
            n106 = To Single Precision Float(number=w207) -> (single precision float=w206:sgl)
            n107 = Initialize Array(w206, w209) -> (w208:sgl[])
          }
          frame Default {
            n108 = expression code="x-1"(w214) -> (w223:u8)
            n109 = expression code="x*2"(w214) -> (w220:u8)
            n110 = Multiply(x=w223, y=w217) -> (x*y=w221:sgl)
            n111 = Subtract(x=w216, y=w217) -> (x-y=w215:sgl)
            n112 = Add(x=w216, y=w221) -> (x+y=w222:sgl)
            n113 = Divide(x=w215, y=w214) -> (x/y=w213:sgl)
            n114 = Divide(x=w222, y=w220) -> (x/y=w219:sgl)
            n115 = for {
              N: w214 -> [_]
              tunnel: w213 -> [w225]
              tunnel: [w224] -> w212 mode=indexing
              i -> [w226]
              n116 = Multiply(x=w225, y=w226) -> (x*y=w224:sgl)
            }
            n117 = To Single Precision Float(number=w218) -> (single precision float=w210:sgl)
            n118 = Compound Arithmetic op=ADD(w210, w219, w212) -> (w211:sgl[])
          }
        }
        n119 = Compound Arithmetic op=ADD(w193, w190, w191) -> (w192:sgl[])
      }
      "X center (um)" <- w121
      n120 = for {
        N: w115 -> [_]
        tunnel: w119 -> [w162]
        tunnel: w118 -> [w161]
        tunnel: w117 -> [w165] mode=indexing
        tunnel: w116 -> [w160]
        tunnel: [w166] -> w114 mode=indexing
        tunnel: w120 -> [w163]
        n121 = expression code="x/2"(w162) -> (w167:sgl)
        n122 = Subtract(x=w163, y=w167) -> (x-y=w164:sgl)
        n123 = case shown="Default" w160 {
          tunnel: w162 -> [_ w178]
          tunnel: w161 -> [_ w179]
          tunnel: w160 -> [w171 w176]
          tunnel: [w170 w173] -> w159
          tunnel: w164 -> [_ w180]
          tunnel: w163 -> [w169 _]
          frame 1 {
            n124 = To Single Precision Float(number=w169) -> (single precision float=w168:sgl)
            n125 = Initialize Array(w168, w171) -> (w170:sgl[])
          }
          frame Default {
            n126 = expression code="x-1"(w176) -> (w185:u8)
            n127 = expression code="x*2"(w176) -> (w182:u8)
            n128 = Multiply(x=w185, y=w179) -> (x*y=w183:sgl)
            n129 = Subtract(x=w178, y=w179) -> (x-y=w177:sgl)
            n130 = Add(x=w178, y=w183) -> (x+y=w184:sgl)
            n131 = Divide(x=w177, y=w176) -> (x/y=w175:sgl)
            n132 = Divide(x=w184, y=w182) -> (x/y=w181:sgl)
            n133 = for {
              N: w176 -> [_]
              tunnel: w175 -> [w187]
              tunnel: [w186] -> w174 mode=indexing
              i -> [w188]
              n134 = Multiply(x=w187, y=w188) -> (x*y=w186:sgl)
            }
            n135 = To Single Precision Float(number=w180) -> (single precision float=w172:sgl)
            n136 = Compound Arithmetic op=ADD(w172, w181, w174) -> (w173:sgl[])
          }
        }
        n137 = Add(x=w159, y=w165) -> (x+y=w166:sgl[])
      }
      n138 = And(x=w108, y=w109) -> (x .and. y?=w107:bool)
      n139 = And(x=w106, y=w105) -> (x .and. y?=w101:bool)
      n140 = And(x=w97, y=w98) -> (x .and. y?=w81:bool)
      n141 = And(x=w96, y=w95) -> (x .and. y?=w83:bool)
      n142 = And(x=w89, y=w90) -> (x .and. y?=w82:bool)
      n143 = case shown="True" w107 {
        tunnel: w141 -> [w292 w296]
        tunnel: w85 -> [w295 _]
        tunnel: w84 -> [w294 _]
        tunnel: [w293 w296] -> w140
        tunnel: w79 -> [w289 _]
        frame False {
          n144 = Reshape Array(w292, w289) -> (w291:sgl[])
          n145 = call-poly <vilib>:"Mean.vi"("X"=w291) -> ("mean"=w290:dbl)  [unwired: 1 out]
          n146 = Initialize Array(w290, w295, w294) -> (w293:dbl[][])
        }
        frame True {
        }
      }
      n147 = case shown="False" w101 {
        tunnel: w102 -> [w282 w288]
        tunnel: w85 -> [w287 _]
        tunnel: w84 -> [w286 _]
        tunnel: [w285 w288] -> w138
        tunnel: w74 -> [w281 _]
        frame False {
          n148 = Reshape Array(w282, w281) -> (w284:sgl[])
          n149 = call-poly <vilib>:"Mean.vi"("X"=w284) -> ("mean"=w283:dbl)  [unwired: 1 out]
          n150 = Initialize Array(w283, w287, w286) -> (w285:dbl[][])
        }
        frame True {
        }
      }
      n151 = case shown="False" w81 {
        tunnel: w88 -> [w274 w280]
        tunnel: w85 -> [w279 _]
        tunnel: w84 -> [w278 _]
        tunnel: [w277 w280] -> w137
        tunnel: w73 -> [w273 _]
        frame False {
          n152 = Reshape Array(w274, w273) -> (w276:sgl[])
          n153 = call-poly <vilib>:"Mean.vi"("X"=w276) -> ("mean"=w275:dbl)  [unwired: 1 out]
          n154 = Initialize Array(w275, w279, w278) -> (w277:dbl[][])
        }
        frame True {
        }
      }
      n155 = case shown="False" w83 {
        tunnel: w87 -> [w266 w272]
        tunnel: w85 -> [w271 _]
        tunnel: w84 -> [w270 _]
        tunnel: [w269 w272] -> w136
        tunnel: w72 -> [w265 _]
        frame False {
          n156 = Reshape Array(w266, w265) -> (w268:sgl[])
          n157 = call-poly <vilib>:"Mean.vi"("X"=w268) -> ("mean"=w267:dbl)  [unwired: 1 out]
          n158 = Initialize Array(w267, w271, w270) -> (w269:dbl[][])
        }
        frame True {
        }
      }
      n159 = case shown="False" w82 {
        tunnel: w86 -> [w259 w264]
        tunnel: w85 -> [w263 _]
        tunnel: w84 -> [w262 _]
        tunnel: [w261 w264] -> w113
        tunnel: w71 -> [w257 _]
        frame False {
          n160 = Reshape Array(w259, w257) -> (w258:sgl[])
          n161 = call-poly <vilib>:"Mean.vi"("X"=w258) -> ("mean"=w260:dbl)  [unwired: 1 out]
          n162 = Initialize Array(w260, w263, w262) -> (w261:dbl[][])
        }
        frame True {
        }
      }
      n163 = Bundle By Name(cluster=w68, "SEM Scan Parameters.X stig"=w140, "SEM Scan Parameters.Y stig"=w138, "SEM Scan Parameters.X aln"=w137, "SEM Scan Parameters.Y aln"=w136, "SEM Scan Parameters.WD (mm)"=w113) -> (w139:T6)
      n164 = local write "Tiled scan inputs"(w139) -> ()
      n165 = Transpose 2D Array(2D array=w62) -> (transposed array=w61:sgl[][])
      n166 = Transpose 2D Array(2D array=w129) -> (transposed array=w67:sgl[][])
      n167 = Divide(x=w48, y=w50) -> (x/y=→"X resolution":sgl[][])
      n168 = Multiply(x=w48, y=w51) -> (x*y=→"X size (V)":dbl[][])
      n169 = Divide(x=w67, y=w50) -> (x/y=→"Y resolution":sgl[][])
      n170 = Transpose 2D Array(2D array=w114) -> (transposed array=→"Y center (um)":sgl[][])
      n171 = Divide(x=w63, y=w66) -> (x/y=→"Tiled image X index":sgl[][])
      n172 = Divide(x=w61, y=w66) -> (x/y=→"Tiled image Y index":sgl[][])
    }
    frame #2 {
      n173 = local read "Tiled scan inputs"() -> (w298:T6)
      n174 = Unbundle By Name(w298) -> ("SEM Scan Parameters.Frames"=w297:u8)
      n175 = for {
        N: w297 -> [_]
        tunnel: w298 -> [w314]
        i -> [w313]
        stop <- w312 stop-if-true
        # "Frame"
        n176 = Unbundle By Name(w314) -> ("SEM Options"=w343:T7, "HW Config"=w342:T8, "Det Info"=w341:T9, "SEM Scan Parameters"=w356:T10, "Focus Index Options"=w305:T11, "File Information"=w340:T12, "Additional Info"=w299:cluster{"Restart flag":u8, "Stage move flag":u8}, "Milling para"=w336:T13)
        n177 = Unbundle By Name(w314) -> ("SEM Options.Detector A"=w324:bool, "SEM Options.Detector B"=w323:bool)
        n178 = Unbundle By Name(w356) -> ("X stig"=w348:sgl[][], "Y stig"=w347:sgl[][], "X aln"=w346:sgl[][], "Y aln"=w345:sgl[][], "Scan rate (Hz)"=w355:u32, "Oversampling"=w354:u32, "Oversampling auto"=w353:bool, "Frame line rampdown ratio"=w352:sgl, "Pixel size (nm)"=w351:sgl, "WD (mm)"=w344:sgl[][])
        n179 = Unbundle By Name(w305) -> ("Keep aspect ratio"=w300:bool, "X Grids"=w304:u8[][], "Y Grids"=w303:u8[][], "Primary X index"=w302:u8[][], "Primary Y index"=w301:u8[][])
        n180 = local read "X resolution"() -> (w350:u32[][])
        n181 = local read "Y resolution"() -> (w349:u32[][])
        n182 = local read "X center (um)"() -> (w339:sgl[][])
        n183 = local read "Y center (um)"() -> (w338:sgl[][])
        n184 = local read "X size (V)"() -> (w337:dbl[][])
        n185 = for {
          tunnel: w355 -> [w402]
          tunnel: w354 -> [w401]
          tunnel: w353 -> [w400]
          tunnel: w352 -> [w399]
          tunnel: w351 -> [w398]
          tunnel: w350 -> [w397] mode=indexing
          tunnel: w349 -> [w396] mode=indexing
          tunnel: w348 -> [w395] mode=indexing
          tunnel: w347 -> [w394] mode=indexing
          tunnel: w346 -> [w393] mode=indexing
          tunnel: w345 -> [w392] mode=indexing
          tunnel: w344 -> [w391] mode=indexing
          tunnel: w343 -> [w390]
          tunnel: w342 -> [w389]
          tunnel: w341 -> [w388]
          tunnel: w340 -> [w387]
          tunnel: w339 -> [w386] mode=indexing
          tunnel: w338 -> [w385] mode=indexing
          tunnel: w337 -> [w384] mode=indexing
          tunnel: w336 -> [w383]
          tunnel: [w381] -> w329 mode=indexing
          tunnel: [w380] -> w328 mode=indexing
          tunnel: [w379] -> w327 mode=indexing
          tunnel: [w378] -> w326 mode=indexing
          tunnel: [w377] -> w332 mode=indexing
          tunnel: [w376] -> w331 mode=indexing
          tunnel: [w375] -> w335 mode=indexing
          tunnel: [w374] -> w334 mode=indexing
          tunnel: [w373] -> w325 mode=indexing
          tunnel: w324 -> [w372]
          tunnel: w323 -> [w371]
          tunnel: [w370] -> w318 mode=concatenating
          tunnel: w313 -> [w369]
          tunnel: [w368] -> w311 mode=indexing
          tunnel: [w367] -> w310 mode=indexing
          tunnel: [w366] -> w306 mode=indexing
          tunnel: [w365] -> w307 mode=indexing
          tunnel: [w364] -> w308 mode=indexing
          tunnel: [w363] -> w309 mode=indexing
          tunnel: w304 -> [w362] mode=indexing
          tunnel: w303 -> [w361] mode=indexing
          tunnel: w302 -> [w360] mode=indexing
          tunnel: w301 -> [w359] mode=indexing
          tunnel: w300 -> [w358]
          tunnel: w299 -> [w357]
          i -> [w382]
          # "Y"
          n186 = for {
            tunnel: w402 -> [w468]
            tunnel: w401 -> [w467]
            tunnel: w400 -> [w466]
            tunnel: w399 -> [w465]
            tunnel: w398 -> [w431]
            tunnel: w397 -> [w425] mode=indexing
            tunnel: w396 -> [w424] mode=indexing
            tunnel: w395 -> [w464] mode=indexing
            tunnel: w394 -> [w463] mode=indexing
            tunnel: w393 -> [w462] mode=indexing
            tunnel: w392 -> [w461] mode=indexing
            tunnel: w391 -> [w434] mode=indexing
            tunnel: w390 -> [w449]
            tunnel: w389 -> [w455]
            tunnel: w388 -> [w454]
            tunnel: w387 -> [w452]
            tunnel: w386 -> [w460] mode=indexing
            tunnel: w385 -> [w459] mode=indexing
            tunnel: w384 -> [w435] mode=indexing
            tunnel: w383 -> [w451]
            tunnel: w382 -> [w430]
            tunnel: [w446] -> w381 mode=indexing
            tunnel: [w445] -> w380 mode=indexing
            tunnel: [w444] -> w379 mode=indexing
            tunnel: [w443] -> w378 mode=indexing
            tunnel: [w441] -> w377 mode=indexing
            tunnel: [w440] -> w376 mode=indexing
            tunnel: [w439] -> w375 mode=indexing
            tunnel: [w438] -> w374 mode=indexing
            tunnel: [w428] -> w373 mode=indexing
            tunnel: w372 -> [w427]
            tunnel: w371 -> [w426]
            tunnel: [w423] -> w370 mode=indexing
            tunnel: w369 -> [w422]
            tunnel: [w420] -> w368 mode=indexing
            tunnel: [w417] -> w367 mode=indexing
            tunnel: [w416] -> w366 mode=indexing
            tunnel: [w415] -> w365 mode=indexing
            tunnel: [w414] -> w364 mode=indexing
            tunnel: [w413] -> w363 mode=indexing
            tunnel: w362 -> [w410] mode=indexing
            tunnel: w361 -> [w409] mode=indexing
            tunnel: w360 -> [w408] mode=indexing
            tunnel: w359 -> [w407] mode=indexing
            tunnel: w358 -> [w406]
            tunnel: w357 -> [w403]
            i -> [w429]
            # "X"
            n187 = local read "ActiveX Container"() -> (w404:refnum<k7>)
            n188 = shared-variable ".\\Zeiss Library.lvlib\\X resolution"(w425) -> ()  [unwired: 1 in, 1 out]
            n189 = Build Array(w430, w429) -> (w448:i32[])
            n190 = Bundle By Name(cluster="SEM Scan Parameters", "X resolution"=w425, "Y resolution"=w424, "X center (um)"=w460, "Y center (um)"=w459, "X size (V)"=w435, "X size auto"=FALSE, "X stig"=w464, "Y stig"=w463, "X aln"=w462, "Y aln"=w461, "Scan rate (Hz)"=w468, "Oversampling"=w467, "Oversampling auto"=w466, "Frame line rampdown ratio"=w465, "Pixel size (nm)"=w431, "WD (mm)"=w434) -> (w453:T5)
            n191 = Bundle By Name(cluster="Focus Index Options", "Keep aspect ratio"=w406, "X Grids"=w410, "Y Grids"=w409, "Primary X index"=w408, "Primary Y index"=w407) -> (w411:T1)
            n192 = flat-sequence {
              tunnel: w430 -> [w477]
              tunnel: w429 -> [w476]
              tunnel: w428 -> [w482]
              tunnel: w427 -> [w470]
              tunnel: w426 -> [w469]
              frame #0 {
                n193 = local read "Det A Img Tiled"() -> (w487:i16[][])
                n194 = shared-variable ".\\Zeiss Library.lvlib\\Det A Img"() -> (w484:i16[][])  [unwired: 1 in, 1 out]
                n195 = shared-variable ".\\Zeiss Library.lvlib\\Det B Img"() -> (w481:i16[][])  [unwired: 1 in, 1 out]
                n196 = local read "Tiled image scale (um/pix)"() -> (w483:sgl)
                n197 = local read "Tiled image Y index"() -> (w489:u16[][])
                n198 = local read "Tiled image X index"() -> (w488:u16[][])
                n199 = local read "Det B Img Tiled"() -> (w478:i16[][])
                n200 = Index Array(array=w489, index (row)=w477, index (col)=w476) -> (element=w474:u16)
                n201 = Index Array(array=w488, index (row)=w477, index (col)=w476) -> (element=w473:u16)
                n202 = Divide(x=w482, y=w483) -> (x/y=w475:dbl)
                n203 = call "2D Array Zoom.vi"("y zoom factor"=w475, "x zoom factor"=w475, "Input 2D Array"=w484) -> ("output array"=w486:dbl[][])  [unwired: 6 in, 2 out]
                n204 = call "2D Array Zoom.vi"("y zoom factor"=w475, "x zoom factor"=w475, "Input 2D Array"=w481) -> ("output array"=w479:dbl[][])  [unwired: 6 in, 2 out]
                n205 = To Word Integer(number=w486) -> (16bit integer=w485:i16[][])
                n206 = To Word Integer(number=w479) -> (16bit integer=w480:i16[][])
                n207 = Replace Array Subset(array=w487, new element=w485, index (row)=w474, index (col)=w473) -> (w471:i16[][])
                n208 = Replace Array Subset(array=w478, new element=w480, index (row)=w474, index (col)=w473) -> (w472:i16[][])
                n209 = case shown="True" w470 {
                  tunnel: w471 -> [_ w491]
                  frame False {
                  }
                  frame True {
                    n210 = local write "Det A Img Tiled"(w491) -> ()
                    n211 = shared-variable ".\\Zeiss Library.lvlib\\Det A Img Tiled"(w491) -> ()  [unwired: 1 in, 1 out]
                  }
                }
                n212 = case shown="True" w469 {
                  tunnel: w472 -> [_ w490]
                  frame False {
                  }
                  frame True {
                    n213 = shared-variable ".\\Zeiss Library.lvlib\\Det B Img Tiled"(w490) -> ()  [unwired: 1 in, 1 out]
                    n214 = local write "Det B Img Tiled"(w490) -> ()
                  }
                }
              }
            }
            n215 = shared-variable ".\\Zeiss Library.lvlib\\Y resolution"(w424) -> ()  [unwired: 1 in, 1 out]
            n216 = call "2D scan Tclk.vi"("ActiveX Container"=w404, "Det Info"=w454, "HW Config"=w455, "Scan Para"=w453, "Focus Index Options"=w411, "File Info"=w452, "Options"=w449, "WatchDog Mode"="WatchDog Mode", "Additional Info"=w403, "Frame"=w422, "Tile index"=w448, "Milling para"=w451) -> ("Image Focus Index Array"=w442:T14, "Info & Status"=w419:T15, "SEM parameters"=w418:T16, "8-bit over scale"=w423:bool[], "FIB parameters"=w450:T17, "Image Focus Index"=w447:T18)  [unwired: 2 in]
            n217 = Unbundle By Name(w442) -> ("A Img Focus Index array"=w441:sgl[][], "B Img Focus Index array"=w440:sgl[][], "C Img Focus Index array"=w439:sgl[][], "D Img Focus Index array"=w438:sgl[][])
            n218 = Unbundle By Name(w418) -> ("Working distance"=w417:sgl, "Stig X"=w416:sgl, "Stig Y"=w415:sgl, "Alignment X"=w414:sgl, "Alignment Y"=w413:sgl)
            n219 = Unbundle By Name(w419) -> ("Decimating factor"=w436:u16)
            n220 = local read "Single scan outputs"() -> (w457:T4)
            n221 = Bundle By Name(cluster=w457, "Image Focus Index Array"=w442, "SEM Status"=w419, "SEM Parameters"=w418, "FIB parameters"=w450, "Image Focus Index"=w447) -> (w421:T4)
            "Single scan outputs" <- w421
            n222 = expression code="x/1000"(w431) -> (w433:sgl)
            n223 = Unbundle By Name(w447) -> ("A Img Focus Index"=w446:sgl, "B Img Focus Index"=w445:sgl, "C Img Focus Index"=w444:sgl, "D Img Focus Index"=w443:sgl)
            n224 = Quotient & Remainder(x=w425, y=w436) -> (floor(x/y)=w437:u32)  [unwired: 1 out]
            n225 = Divide(x=w425, y=w437) -> (x/y=w432:dbl)
            n226 = Unbundle By Name(w421) -> ("SEM Status.SEM Spec. I (nA)"=w420:sgl)
            n227 = Multiply(x=w433, y=w432) -> (x*y=w428:dbl)
          }
        }
        "Low res scale Tiled (um/pix)" <- w325
        "SEM Spec. I Tiled (nA)" <- w311
        "WD Tiled" <- w310
        "Stig X Tiled" <- w306
        "Stig Y Tiled" <- w307
        "Aln X Tiled" <- w308
        "Aln Y Tiled" <- w309
        n228 = Bundle("A Img Focus Index array"=w332, "B Img Focus Index array"=w331, "C Img Focus Index array"=w335, "D Img Focus Index array"=w334) -> (→"Image Focus Index Array Tiled":T2)  [unwired: 1 in]
        n229 = Bundle(w329, w328, w327, w326) -> (→"Image Focus Index Tiled":cluster{sgl[][], sgl[][], sgl[][], sgl[][]})  [unwired: 1 in]
        n230 = Index Array(array=w318, index (col) #1=0 ("index (row)"), index (col) #2=1 ("index (row)")) -> (element #1=w319:bool[], element #2=w320:bool[])  [unwired: 2 in]
        n231 = And Array Elements(Boolean array=w319) -> (logical AND=w317:bool)
        n232 = And Array Elements(Boolean array=w320) -> (logical AND=w315:bool)
        n233 = Build Array(w317, w315) -> (→"8-bit over scale":bool[])
        n234 = shared-variable "My Computer\\Zeiss Library.lvlib\\Stop"() -> (w312:bool)  [unwired: 1 in, 1 out]
      }
    }
    frame #3 {
      n235 = shared-variable "My Computer\\Zeiss Library.lvlib\\Machine Type"() -> (w492:u8)  [unwired: 1 in, 1 out]
      n236 = case shown="2" w492 {
        frame 0, Default {
          n237 = local read "Tiled scan inputs"() -> (w494:T6)
          n238 = Unbundle By Name(w494) -> ("HW Config.Eanable COM"=w493:bool)
          n239 = case shown="True" w493 {
            tunnel: w494 -> [_ w510]
            frame False {
            }
            frame True {
              n240 = Unbundle By Name(w510) -> ("HW Config.COM port"=w509:refnum<visa-resource-name>, "SEM Scan Parameters.Y tiles"=w508:u8, "SEM Scan Parameters.X tiles"=w507:u8)  [unwired: 5 out]
              n241 = local read "Stig X Tiled"() -> (w499:sgl[][])
              n242 = local read "Stig Y Tiled"() -> (w498:sgl[][])
              n243 = expression code="(x-1)/2"(w508) -> (w502:u8)
              n244 = expression code="(x-1)/2"(w507) -> (w501:u8)
              n245 = Index Array(array=w499, index (row)=w502, index (col)=w501) -> (element=w506:sgl)
              n246 = Index Array(array=w498, index (row)=w502, index (col)=w501) -> (element=w505:sgl)
              n247 = Format Into String(format string="stim %g %g", w506, w505) -> (resulting string=w522:string)  [unwired: 2 in, 1 out]
              n248 = local read "Aln X Tiled"() -> (w497:sgl[][])
              n249 = local read "Aln Y Tiled"() -> (w496:sgl[][])
              n250 = call "Remcon32 command.vi"("Initialization"=TRUE, "SEM command"=w522, "COM port in"=w509) -> ("error out"=w513:errorcluster, "COM port out"=w514:refnum<visa-resource-name>)  [unwired: 2 in, 5 out]
              n251 = Index Array(array=w497, index (row)=w502, index (col)=w501) -> (element=w504:sgl)
              n252 = Index Array(array=w496, index (row)=w502, index (col)=w501) -> (element=w503:sgl)
              n253 = Format Into String(format string="aaln %g %g", w504, w503) -> (resulting string=w520:string)  [unwired: 2 in, 1 out]
              n254 = local read "WD Tiled"() -> (w495:sgl[][])
              n255 = call "Remcon32 command.vi"("error in"=w513, "SEM command"=w520, "COM port in"=w514) -> ("error out"=w511:errorcluster, "COM port out"=w512:refnum<visa-resource-name>)  [unwired: 2 in, 5 out]
              n256 = Index Array(array=w495, index (row)=w502, index (col)=w501) -> (element=w500:sgl)
              n257 = Format Into String(format string="focs %g", w500) -> (resulting string=w518:string)  [unwired: 2 in, 1 out]
              n258 = call "Remcon32 command.vi"("Close session"=TRUE, "error in"=w511, "SEM command"=w518, "COM port in"=w512) -> ()  [unwired: 1 in, 7 out]
            }
          }
        }
        frame 2 {
          n259 = local read "Tiled scan inputs"() -> (w552:T6)
          n260 = Unbundle By Name(w552) -> ("SEM Scan Parameters.Y tiles"=w551:u8, "SEM Scan Parameters.X tiles"=w550:u8)  [unwired: 5 out]
          n261 = local read "Stig X Tiled"() -> (w547:sgl[][])
          n262 = local read "Stig Y Tiled"() -> (w546:sgl[][])
          n263 = expression code="(x-1)/2"(w551) -> (w549:u8)
          n264 = expression code="(x-1)/2"(w550) -> (w548:u8)
          n265 = Index Array(array=w547, index (row)=w549, index (col)=w548) -> (element=w532:sgl)
          n266 = Index Array(array=w546, index (row)=w549, index (col)=w548) -> (element=w526:sgl)
          n267 = local read "Aln X Tiled"() -> (w545:sgl[][])
          n268 = local read "Aln Y Tiled"() -> (w544:sgl[][])
          n269 = call "SmartSEM Remote API set float.vi"("vValue"=w532, "lpszParam"="AP_STIG_X" ("lpszCommand"), "ActiveX Container"="ActiveX Container") -> ("error out"=w539:errorcluster, "reference out"=w540:refnum<k7>)  [unwired: 7 in]
          n270 = Index Array(array=w545, index (row)=w549, index (col)=w548) -> (element=w537:sgl)
          n271 = Index Array(array=w544, index (row)=w549, index (col)=w548) -> (element=w527:sgl)
          n272 = local read "WD Tiled"() -> (w543:sgl[][])
          n273 = call "SmartSEM Remote API set float.vi"("error in"=w539, "vValue"=w537, "lpszParam"="AP_APERTURE_ALIGN_X" ("lpszCommand"), "ActiveX Container"=w540) -> ("error out"=w535:errorcluster, "reference out"=w536:refnum<k7>)  [unwired: 6 in]
          n274 = Index Array(array=w543, index (row)=w549, index (col)=w548) -> (element=w542:sgl)
          n275 = expression code="x/1000"(w542) -> (w533:sgl)
          n276 = call "SmartSEM Remote API set float.vi"("error in"=w535, "vValue"=w533, "lpszParam"="AP_WD" ("lpszCommand"), "ActiveX Container"=w536) -> ("error out"=w523:errorcluster, "reference out"=w524:refnum<k7>)  [unwired: 6 in]
          n277 = call "SmartSEM Remote API set float.vi"("error in"=w523, "vValue"=w526, "lpszParam"="AP_STIG_Y" ("lpszCommand"), "ActiveX Container"=w524) -> ("error out"=w529:errorcluster, "reference out"=w530:refnum<k7>)  [unwired: 6 in]
          n278 = call "SmartSEM Remote API set float.vi"("error in"=w529, "vValue"=w527, "lpszParam"="AP_APERTURE_ALIGN_Y" ("lpszCommand"), "ActiveX Container"=w530) -> ()  [unwired: 6 in, 2 out]
        }
      }
    }
  }
